vi "duplicated_data.vi"() -> ()   [LabVIEW 2021]
panel:
  out "result b (=0.5)":dbl
  out "result a (=4)":dbl
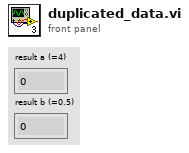
[diagram p1: front panel]
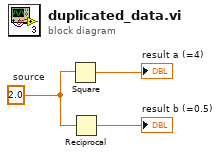
[diagram p0: block diagram]
diagram:
  w3 = 2.0  # source
  n1 = Square(x=w3) -> (x^2=→"result a (=4)":dbl)
  n2 = Reciprocal(x=w3) -> (1/x=→"result b (=0.5)":dbl)
